vi "Readstatus.vi"(8 "error in (no error)":errorcluster, 11 "object in":refnum<class "status Message.lvclass">) -> (0 "error out":errorcluster, 2 "status":T1, 3 "object out":refnum<class "status Message.lvclass">)   [LabVIEW 2018, in "ClientMessaging.lvlib" / "status Message.lvclass"]
uses:
  status Message.lvclass
  Status Content.ctl
  status Message.lvclass/status Message.ctl
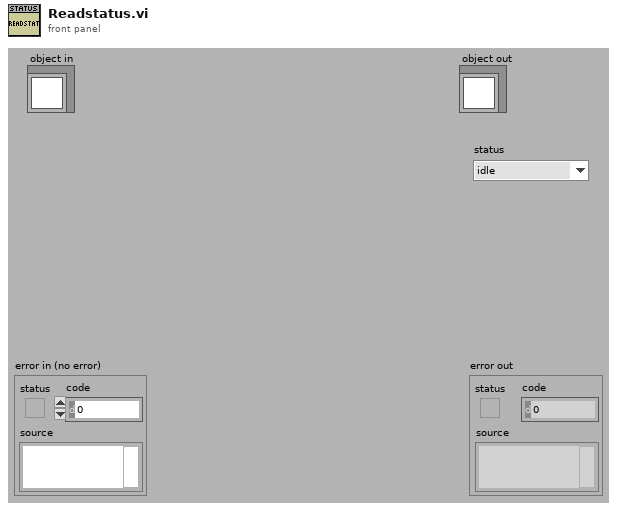
[diagram p1: front panel]
types:
  T1 = typedef "ClientMessaging.lvlib/status Message.lvclass/Status Content.ctl" = enum16{"idle", "busy", "starting"}
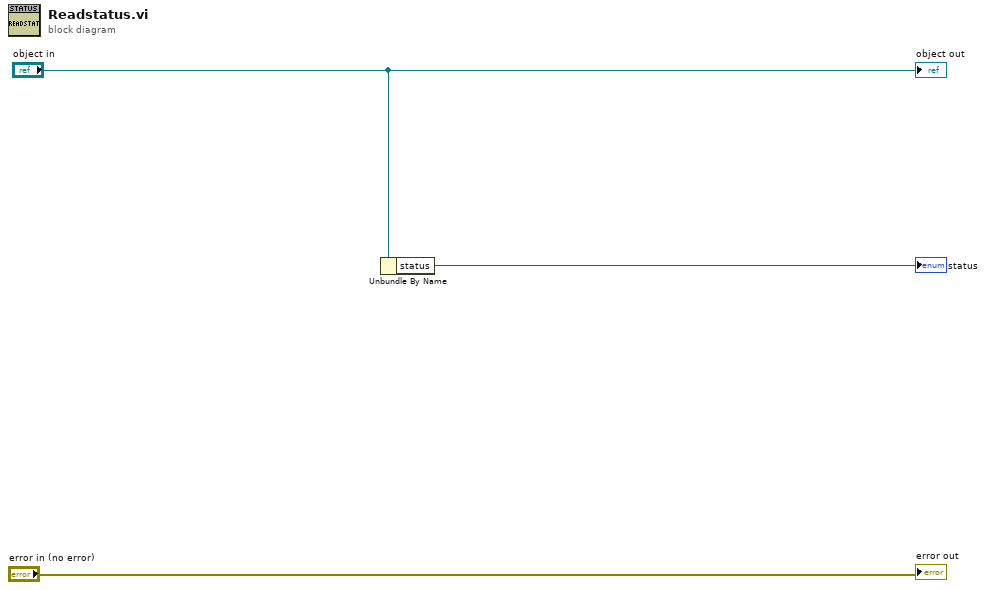
[diagram p0: block diagram]
diagram:
  n1 = Unbundle By Name("object in") -> ("status"=→"status":T1)
  "error out" <- "error in (no error)"
  "object out" <- "object in"
